vi "Cmd objectRepository.vi"(0 "command reference":T2, 1 "method":T3, 2 "occurrence":refnum<k4>, 5 "flags in":i32 format="%.0x", 7 "name in":string, 9 "classDataIn":T4, 11 "error in (no error)":errorcluster) -> (4 "command reference out":T2, 6 "flags out":i32 format="%.0x", 8 "name out":string, 10 "classDataOut":T4, 13 "stats":T1 {"time" format="%<%I:%M:%S%2u %p>T"}, 14 "[references out]":i32[](array[numeric]) format="%.0x", 15 "error out":errorcluster)   [LabVIEW 2012, in "NI_Database_API_64.lvlib"]
doc: "This VI manages objects of the <B>Command</B> class.\n\n[GOOP 1.0/1.0]"
uses:
  NI_Database_API_64.lvlib
  Cmd ObjectReference.ctl
  Cmd DataMembers.ctl
  Connection.llb/Conn ObjectReference.ctl
  <vilib>/Utility/_goopsup.llb/GOOP Object Repository Method.ctl
  <vilib>/Utility/_goopsup.llb/GOOP Object Repository Statistics.ctl
panel:
  in  "debugging":bool
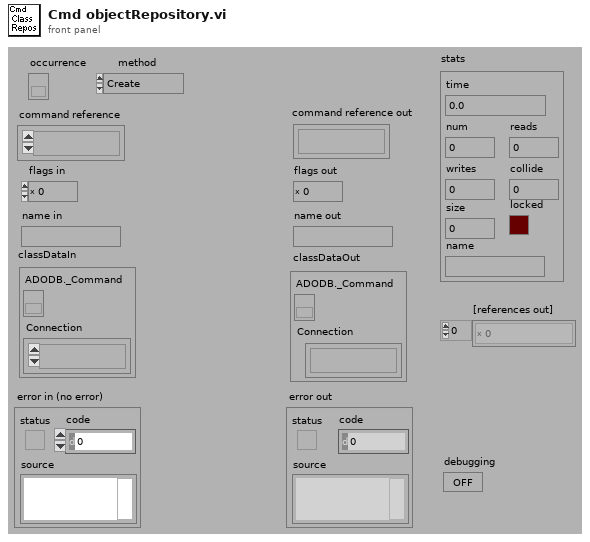
[diagram p1: front panel]
types:
  T1 = typedef "GOOP Object Repository Statistics.ctl" = cluster{"time":dbl, "num":u32, "reads":u32, "writes":u32, "collide":u32, "size":u32, "name":string, "locked":bool}
  T2 = typedef "NI_Database_API_64.lvlib/Cmd ObjectReference.ctl" = refnum<k1>
  T3 = typedef "GOOP Object Repository Method.ctl" = enum16{"Create", "GetCopy", "GetModify", "Set", "Destroy", "Create Static", "Get All Refs", "Reset", "Get Statistics"}
  T4 = typedef "NI_Database_API_64.lvlib/Cmd DataMembers.ctl" = cluster{"ADODB._Command":refnum<k7>, "Connection":T5}
  T5 = typedef "NI_Database_API_64.lvlib/Conn ObjectReference.ctl" = refnum<k1>
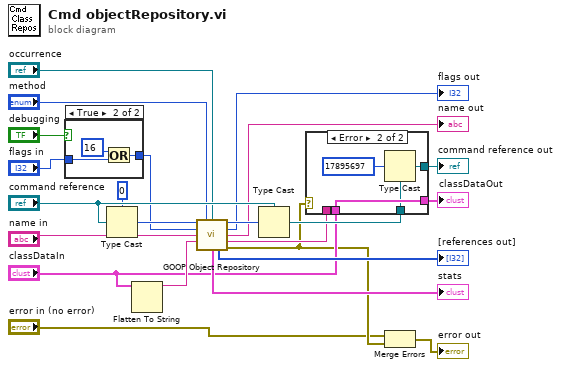
[diagram p0: block diagram]
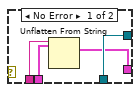
[diagram p2: hidden frame]
diagram:
  n1 = case shown="True" "debugging" {
    tunnel: "flags in" -> [w24 w27]
    tunnel: [w24 w26] -> w11
    frame False {
    }
    frame True {
      n2 = Or(x=16, y=w27) -> (x .or. y?=w26:i32)
    }
  }
  n3 = Type Cast(type=0 ("object ref in"), x="command reference") -> (*(type *) &x=w20:i32)
  n4 = Flatten To String(anything="classDataIn") -> (data string=w15:string)  [unwired: 1 in, 4 out]
  n5 = call <vilib>:"GOOP Object Repository.vi"("object ref in"=w20, "method"="method", "occurrence"="occurrence", "flags in"=w11, "name in"="name in", "object data in"=w15) -> ("object ref out"=w18:i32, "flags out"=→"flags out":i32, "name out"=→"name out":string, "object data out"=w5:string, "stats"=→"stats":T1, "[references out]"=→"[references out]":i32[], "error out"=w2:errorcluster)  [unwired: 1 in, 2 out]
  n6 = Type Cast(type="command reference", x=w18) -> (*(type *) &x=w7:T2)
  n7 = case shown="Error" w2 {
    tunnel: w7 -> [w31 w33]
    tunnel: [w31 w34] -> w23
    tunnel: "classDataIn" -> [w30 w35]
    tunnel: w5 -> [w29 _]
    tunnel: [w28 w35] -> w4
    frame No Error {
      n8 = Unflatten From String(type=w30, binary string=w29) -> (value=w28:T4)  [unwired: 1 in, 4 out]
    }
    frame Error {
      n9 = Type Cast(type=w33, x=17895697) -> (*(type *) &x=w34:T2)
    }
  }
  "command reference out" <- w23
  "classDataOut" <- w4
  n10 = Merge Errors("error in (no error)", w2) -> (→"error out":errorcluster)
